vi "SaveLoop.vi"(8 "error in (no error)":errorcluster, 10 "Queue cluster":T1, 11 "ctrls":T2) -> ()   [LabVIEW 2017]
uses:
  controls_main.ctl
  QueueCluster.ctl
  EventQueueCluster.ctl
  EventMessage.ctl
  MeasureQueue.ctl
  MeasureMessage.ctl
  HardwareQueueCluster.ctl
  hardwareMessage.ctl
  GUIQueueCluster.ctl
  GUIMessage.ctl
  SaveQueueCluster.ctl
  SaveMessage.ctl
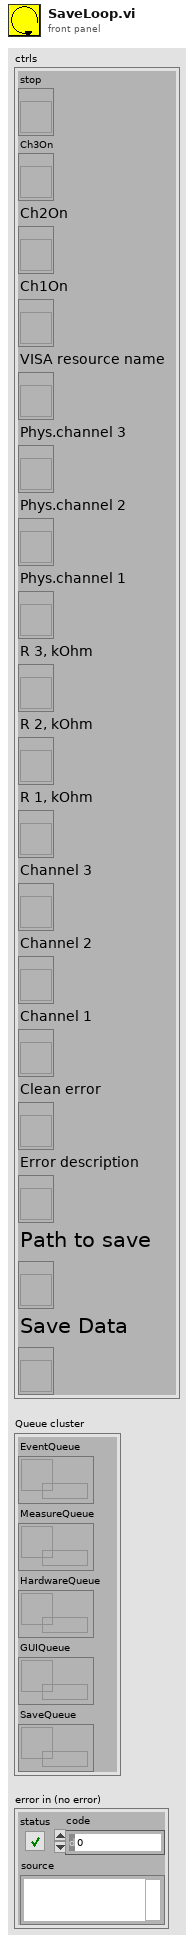
[diagram p1: front panel]
types:
  T1 = typedef "QueueCluster.ctl" = cluster{"EventQueue":refnum<queue>, "MeasureQueue":refnum<queue>, "HardwareQueue":refnum<queue>, "GUIQueue":refnum<queue>, "SaveQueue":refnum<queue>}
  T2 = typedef "controls_main.ctl" = cluster{"stop":refnum<vi>, "Ch3On":refnum<vi>, "Ch2On":refnum<vi>, "Ch1On":refnum<vi>, "VISA resource name":refnum<vi>, "Phys.channel 3":refnum<vi>, "Phys.channel 2":refnum<vi>, "Phys.channel 1":refnum<vi>, "R 3, kOhm":refnum<vi>, "R 2, kOhm":refnum<vi>, "R 1, kOhm":refnum<vi>, "Channel 3":refnum<vi>, "Channel 2":refnum<vi>, "Channel 1":refnum<vi>, "Clean error":refnum<vi>, "Error description":refnum<vi>, "Path to save":refnum<vi>, "Save Data":refnum<vi>}
  T3 = typedef "GUIQueueCluster.ctl" = cluster{"GUIMessage":T4, "NumericValue":dbl, "String":string}
  T4 = typedef "GUIMessage.ctl" = enum16{"StopSave", "Channel1Value", "Channel2Value", "Channel3Value", "ErrorSource", "CleanError", "StartChannel1", "StartChannel2", "StartChannel3", "StopChannel1", "StopChannel2", "StopChannel3", "Halt"}
  T5 = enum16{"open", "replace", "create", "open or create", "replace or create", "replace or create with confirmation"}
  T6 = typedef "SaveQueueCluster.ctl" = cluster{"Save message":T7, "NumericValue":dbl, "String":string}
  T7 = typedef "SaveMessage.ctl" = enum16{"StartSaving", "StopSaving", "Ch1Value", "Ch2Value", "Ch3Value", "Error", "WriteFile", "Halt"}
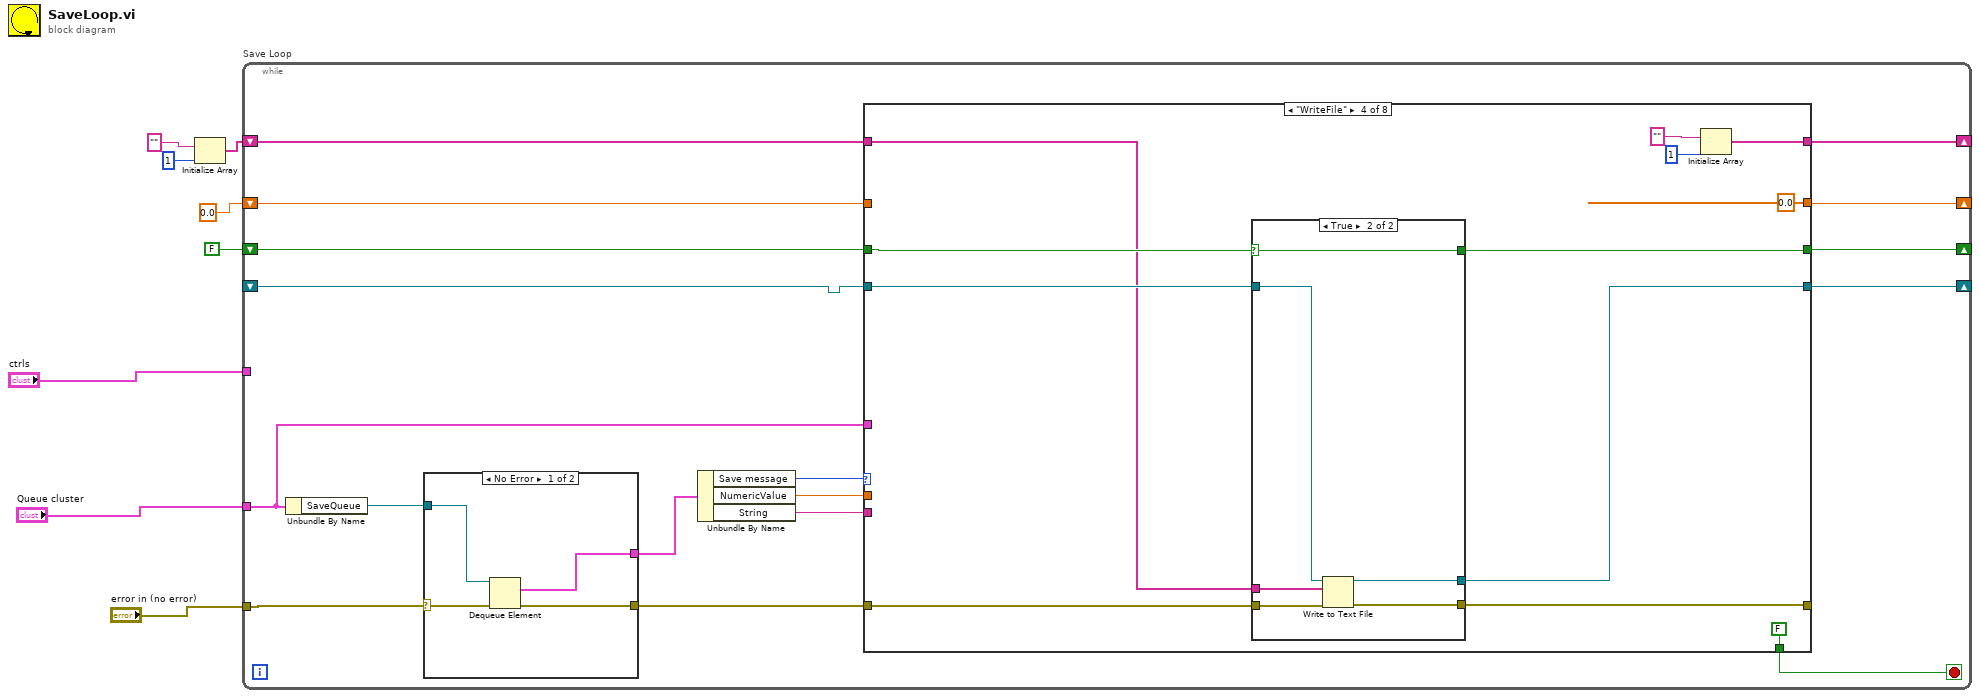
[diagram p0: block diagram]
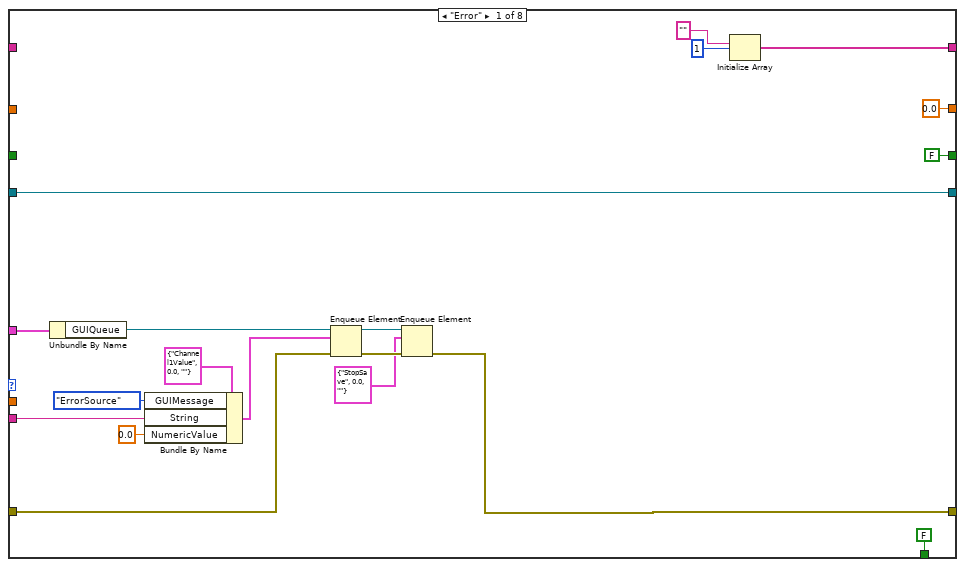
[diagram p2: hidden frame]
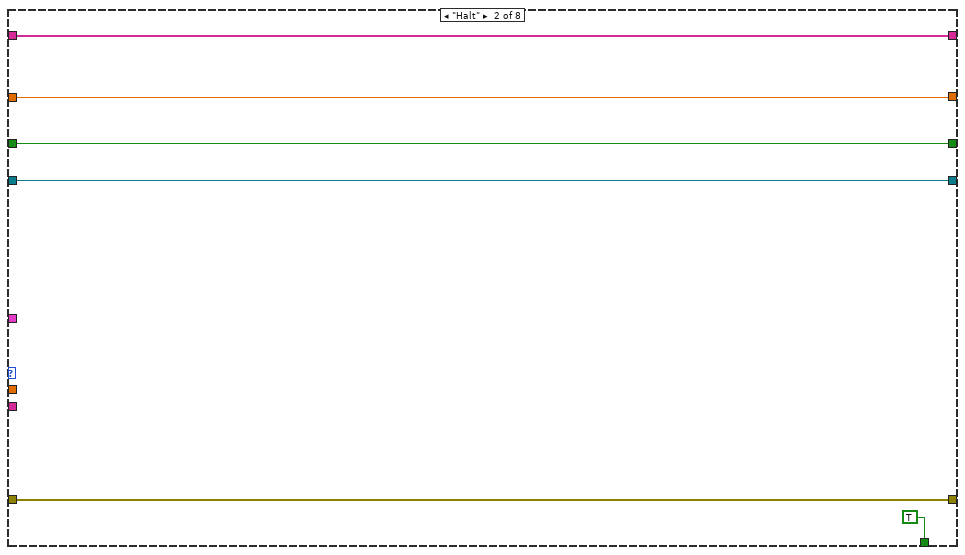
[diagram p3: hidden frame]
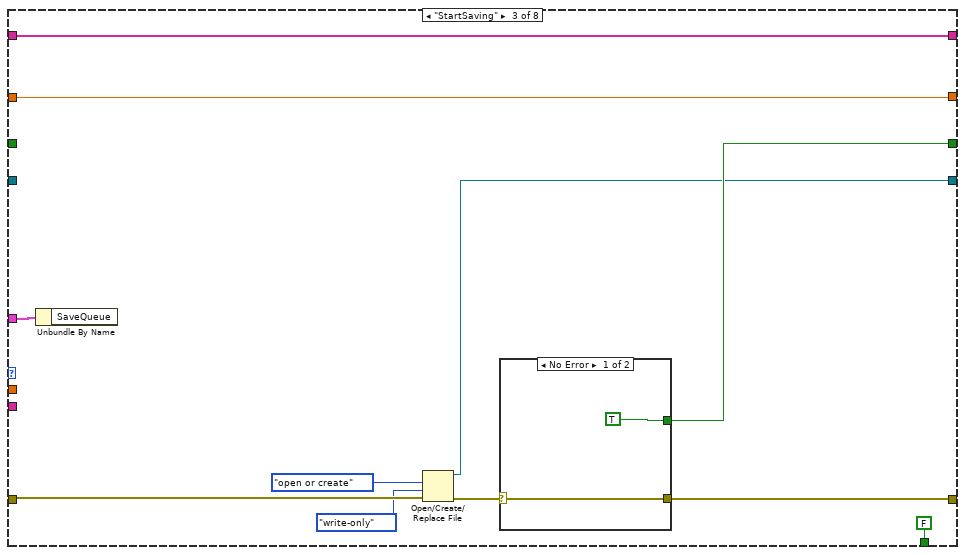
[diagram p4: hidden frame]
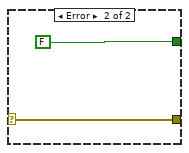
[diagram p5: hidden frame]
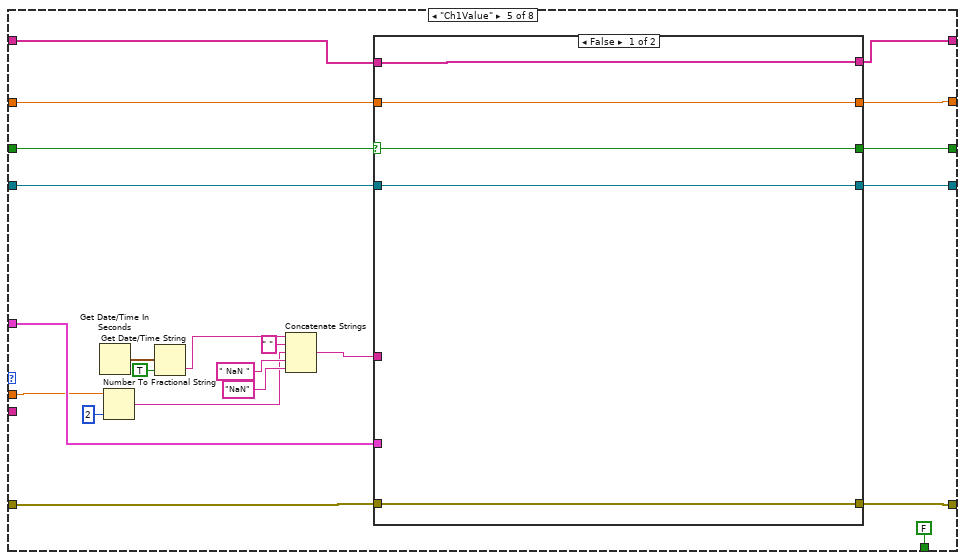
[diagram p7: hidden frame]
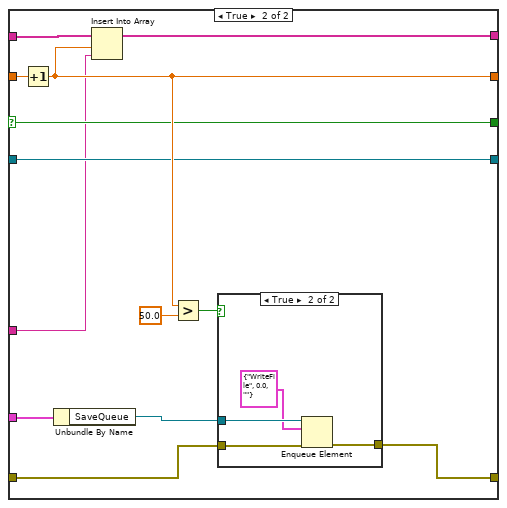
[diagram p8: hidden frame]
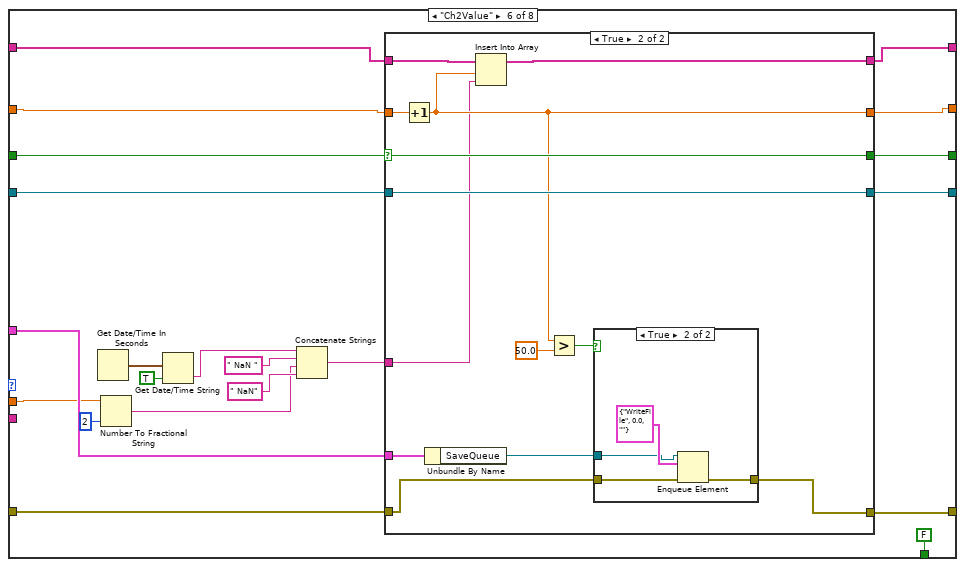
[diagram p10: hidden frame]
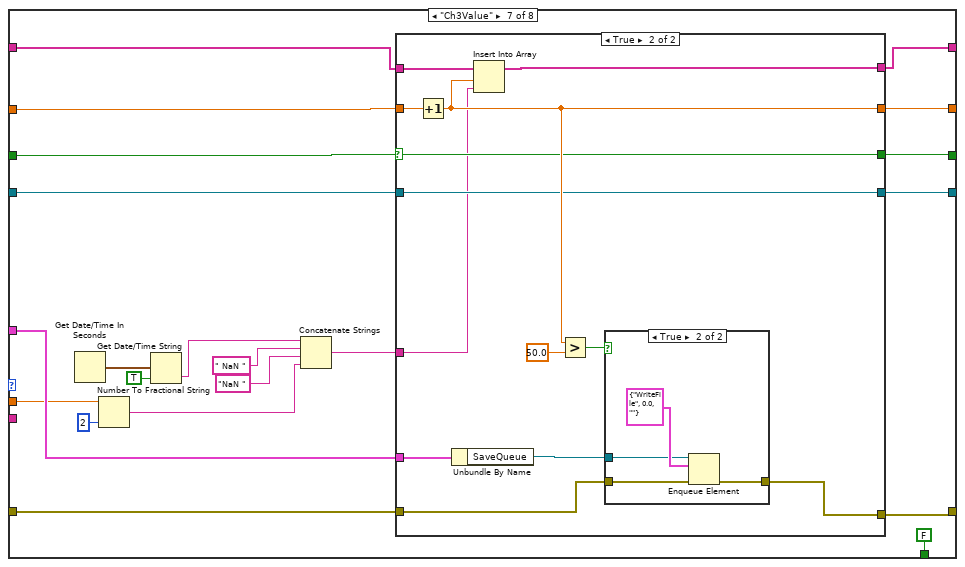
[diagram p13: hidden frame]
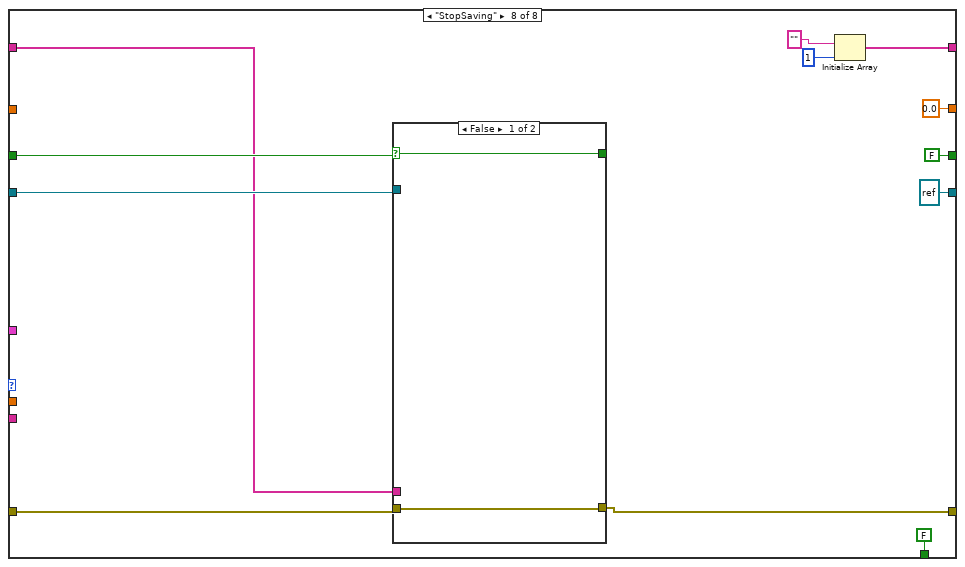
[diagram p16: hidden frame]
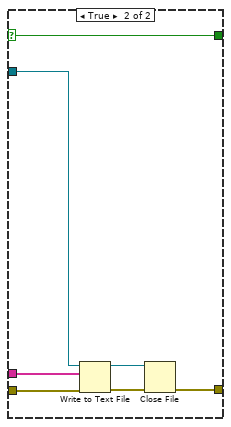
[diagram p17: hidden frame]
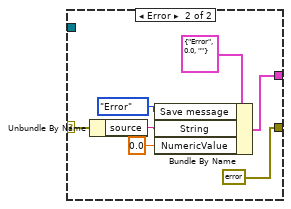
[diagram p18: hidden frame]
diagram:
  n1 = Initialize Array("" ("element"), 1 ("dimension size")) -> (w4:string[])
  n2 = while "Save Loop" {
    tunnel: "Queue cluster" -> [w20]
    tunnel: "ctrls" -> [_]
    tunnel: "error in (no error)" -> [w25]
    shift-right: [w14] -> _
    shift-left: 0.0 -> [w16]
    shift-right: [w15] -> _
    shift-left: w4 -> [w17]
    shift-right: [w12] -> _
    shift-left: FALSE -> [w13]
    shift-right: [w11] -> _
    shift-left: _ -> [w10]
    stop <- w9 stop-if-true
    n3 = Unbundle By Name(w20) -> ("SaveQueue"=w24:refnum<queue>)
    n4 = case shown="No Error" w25 {
      selector: w25 -> [w244 w248]
      tunnel: w24 -> [w243 _]
      tunnel: [w242 w246] -> w23
      tunnel: [w241 errorcluster {"status"=FALSE, "code"=0, "source"=""} ("error out")] -> w21
      frame No Error {
        n5 = Dequeue Element(queue=w243, error in (no error)=w244) -> (element=w242:T6, error out=w241:errorcluster)  [unwired: 1 in, 2 out]
      }
      frame Error {
        n6 = Unbundle By Name(w248) -> ("source"=w247:string)
        n7 = Bundle By Name(cluster=T6 {"Save message"=enum."Error", "NumericValue"=0.0, "String"=""} ("SaveQueueCluster"), "Save message"=SaveMessage."Error", "String"=w247, "NumericValue"=0.0) -> (w246:T6)
      }
    }
    n8 = Unbundle By Name(w23) -> ("Save message"=w22:T7, "NumericValue"=w18:dbl, "String"=w19:string)
    n9 = case shown="\"WriteFile\"" w22 {
      tunnel: w21 -> [w42 w50 w61 w72 w105 w151 w190 w229]
      tunnel: w20 -> [w44 _ w54 _ w104 w146 w191 _]
      tunnel: w19 -> [w39 _ _ _ _ _ _ _]
      tunnel: [w33 w50 w53 w71 w103 w150 w185 w226] -> _
      tunnel: w18 -> [_ _ _ _ w90 w135 w179 _]
      tunnel: w17 -> [_ w48 w55 w69 w107 w148 w195 w228]
      tunnel: w16 -> [_ w47 w56 _ w101 w142 w193 _]
      tunnel: [w30 w48 w55 w75 w106 w149 w194 w222] -> w15
      tunnel: [0.0 w47 w56 0.0 w100 w141 w189 0.0] -> w14
      tunnel: w13 -> [_ w46 _ w70 w102 w147 w192 w231]
      tunnel: [FALSE w46 w57 w67 w99 w145 w186 FALSE] -> w12
      tunnel: [w27 w45 w52 w68 w97 w143 w187 refnum<file> refnum ("refnum out")] -> w11
      tunnel: w10 -> [w27 w45 _ w73 w98 w144 w188 w230]
      tunnel: [FALSE TRUE FALSE FALSE FALSE FALSE FALSE FALSE] -> w9
      frame "Error" {
        n10 = Unbundle By Name(w44) -> ("GUIQueue"=w43:refnum<queue>)
        n11 = Bundle By Name(cluster=T3 {"GUIMessage"=enum."Channel1Value", "NumericValue"=0.0, "String"=""} ("element"), "GUIMessage"=GUIMessage."ErrorSource", "String"=w39, "NumericValue"=0.0) -> (w37:T3)
        n12 = Enqueue Element(queue=w43, element=w37, error in (no error)=w42) -> (queue out=w36:refnum<queue>, error out=w35:errorcluster)  [unwired: 1 in, 1 out]
        n13 = Enqueue Element(queue=w36, element=T3 {"GUIMessage"=enum."StopSave", "NumericValue"=0.0, "String"=""}, error in (no error)=w35) -> (error out=w33:errorcluster)  [unwired: 1 in, 2 out]
        n14 = Initialize Array("" ("element"), 1 ("dimension size")) -> (w30:string[])
      }
      frame "Halt" {
      }
      frame "StartSaving" {
        n15 = Unbundle By Name(w54) -> ()  [unwired: 1 out]
        n16 = Open/Create/Replace File(error in=w61, operation (0:open)=T5."open or create", access (0:read/write)=enum16{"read/write", "read-only", "write-only"}."write-only") -> (refnum out=w52:refnum<file>, error out=w58:errorcluster)  [unwired: 3 in, 1 out]
        n17 = case shown="No Error" w58 {
          selector: w58 -> [w63 w65]
          tunnel: [TRUE FALSE] -> w57
          tunnel: [w63 w65] -> w53
          frame No Error {
          }
          frame Error {
          }
        }
      }
      frame "WriteFile" {
        n18 = case shown="True" w70 {
          selector: w70 -> [w80 w81]
          tunnel: w73 -> [w79 w84]
          tunnel: w72 -> [w78 w86]
          tunnel: [w78 w85] -> w71
          tunnel: w69 -> [_ w83]
          tunnel: [w79 w82] -> w68
          tunnel: [w80 w81] -> w67
          frame False {
          }
          frame True {
            n19 = Write to Text File(file (use dialog)=w84, text=w83, error in=w86) -> (refnum out=w82:refnum<file>, error out=w85:errorcluster)  [unwired: 1 in, 1 out]
          }
        }
        n20 = Initialize Array("" ("element"), 1 ("dimension size")) -> (w75:string[])
      }
      frame "Ch1Value" {
        n21 = Get Date/Time In Seconds() -> (seconds since 1Jan1904=w108:timestamp)
        n22 = Number To Fractional String(number=w90, precision (6)=i16 2) -> (F-format string=w89:string)  [unwired: 2 in]
        n23 = Get Date/Time String(seconds (now)=w108, want seconds? (F)=TRUE) -> (time string=w92:string)  [unwired: 1 in, 1 out]
        n24 = Concatenate Strings(w92, " " ("string"), w89, " NaN " ("element"), "NaN" ("element")) -> (w93:string)
        n25 = case shown="False" w102 {
          selector: w102 -> [w110 w116]
          tunnel: w107 -> [w113 w126]
          tunnel: [w113 w123] -> w106
          tunnel: w105 -> [w112 w120]
          tunnel: w104 -> [_ w122]
          tunnel: [w112 w119] -> w103
          tunnel: w101 -> [w111 w118]
          tunnel: [w111 w117] -> w100
          tunnel: [w110 w116] -> w99
          tunnel: w98 -> [w109 w115]
          tunnel: [w109 w115] -> w97
          tunnel: w93 -> [_ w114]
          frame False {
          }
          frame True {
            n26 = Increment(x=w118) -> (x+1=w117:dbl)
            n27 = Unbundle By Name(w122) -> ("SaveQueue"=w121:refnum<queue>)
            n28 = Insert Into Array(array=w126, index=w117, new element=w114) -> (w123:string[])
            n29 = Greater?(x=w117, y=50.0) -> (0:w125:bool)
            n30 = case shown="True" w125 {
              tunnel: w121 -> [_ w131]
              tunnel: w120 -> [w127 w130]
              tunnel: [w127 w128] -> w119
              frame False {
              }
              frame True {
                n31 = Enqueue Element(queue=w131, element=T6 {"Save message"=enum."WriteFile", "NumericValue"=0.0, "String"=""}, error in (no error)=w130) -> (error out=w128:errorcluster)  [unwired: 1 in, 2 out]
              }
            }
          }
        }
      }
      frame "Ch2Value" {
        n32 = Get Date/Time In Seconds() -> (seconds since 1Jan1904=w152:timestamp)
        n33 = Number To Fractional String(number=w135, precision (6)=i16 2) -> (F-format string=w133:string)  [unwired: 2 in]
        n34 = Get Date/Time String(seconds (now)=w152, want seconds? (F)=TRUE) -> (time string=w139:string)  [unwired: 1 in, 1 out]
        n35 = Concatenate Strings(w139, " NaN " ("element"), w133, " NaN" ("element")) -> (w136:string)
        n36 = case shown="True" w147 {
          selector: w147 -> [w154 w162]
          tunnel: [w156 w168] -> w149
          tunnel: [w157 w166] -> w150
          tunnel: w151 -> [w157 w163]
          tunnel: w148 -> [w156 w165]
          tunnel: w146 -> [_ w164]
          tunnel: [w154 w162] -> w145
          tunnel: w144 -> [w155 w161]
          tunnel: [w155 w161] -> w143
          tunnel: w142 -> [w153 w160]
          tunnel: [w153 w159] -> w141
          tunnel: w136 -> [_ w158]
          frame False {
          }
          frame True {
            n37 = Increment(x=w160) -> (x+1=w159:dbl)
            n38 = Unbundle By Name(w164) -> ("SaveQueue"=w167:refnum<queue>)
            n39 = Insert Into Array(array=w165, index=w159, new element=w158) -> (w168:string[])
            n40 = Greater?(x=w159, y=50.0) -> (0:w170:bool)
            n41 = case shown="True" w170 {
              tunnel: w167 -> [_ w172]
              tunnel: [w171 w174] -> w166
              tunnel: w163 -> [w171 w173]
              frame False {
              }
              frame True {
                n42 = Enqueue Element(queue=w172, element=T6 {"Save message"=enum."WriteFile", "NumericValue"=0.0, "String"=""}, error in (no error)=w173) -> (error out=w174:errorcluster)  [unwired: 1 in, 2 out]
              }
            }
          }
        }
      }
      frame "Ch3Value" {
        n43 = Get Date/Time In Seconds() -> (seconds since 1Jan1904=w196:timestamp)
        n44 = Number To Fractional String(number=w179, precision (6)=i16 2) -> (F-format string=w177:string)  [unwired: 2 in]
        n45 = Get Date/Time String(seconds (now)=w196, want seconds? (F)=TRUE) -> (time string=w183:string)  [unwired: 1 in, 1 out]
        n46 = Concatenate Strings(w183, " NaN " ("element"), "NaN " ("element"), w177) -> (w180:string)
        n47 = case shown="True" w192 {
          selector: w192 -> [w198 w203]
          tunnel: w195 -> [w201 w214]
          tunnel: [w201 w211] -> w194
          tunnel: [w200 w209] -> w185
          tunnel: w193 -> [w199 w206]
          tunnel: w191 -> [_ w208]
          tunnel: w190 -> [w200 w207]
          tunnel: [w199 w205] -> w189
          tunnel: w188 -> [w197 w204]
          tunnel: [w197 w204] -> w187
          tunnel: [w198 w203] -> w186
          tunnel: w180 -> [_ w202]
          frame False {
          }
          frame True {
            n48 = Increment(x=w206) -> (x+1=w205:dbl)
            n49 = Unbundle By Name(w208) -> ("SaveQueue"=w210:refnum<queue>)
            n50 = Insert Into Array(array=w214, index=w205, new element=w202) -> (w211:string[])
            n51 = Greater?(x=w205, y=50.0) -> (0:w213:bool)
            n52 = case shown="True" w213 {
              tunnel: w210 -> [_ w217]
              tunnel: [w215 w218] -> w209
              tunnel: w207 -> [w215 w216]
              frame False {
              }
              frame True {
                n53 = Enqueue Element(queue=w217, element=T6 {"Save message"=enum."WriteFile", "NumericValue"=0.0, "String"=""}, error in (no error)=w216) -> (error out=w218:errorcluster)  [unwired: 1 in, 2 out]
              }
            }
          }
        }
      }
      frame "StopSaving" {
        n54 = case shown="False" w231 {
          selector: w231 -> [w233 w237]
          tunnel: w230 -> [_ w239]
          tunnel: w229 -> [w232 w240]
          tunnel: [w232 w234] -> w226
          tunnel: w228 -> [_ w238]
          tunnel: [w233 w237] -> _
          frame False {
          }
          frame True {
            n55 = Write to Text File(file (use dialog)=w239, text=w238, error in=w240) -> (refnum out=w236:refnum<file>, error out=w235:errorcluster)  [unwired: 1 in, 1 out]
            n56 = Close File(refnum=w236, error in=w235) -> (error out=w234:errorcluster)  [unwired: 1 out]
          }
        }
        n57 = Initialize Array("" ("element"), 1 ("dimension size")) -> (w222:string[])
      }
    }
  }
